vi "ReadSpreadsheetFile.vi"(0 "file (use dialog)":path) -> (1 "Array":dbl[][](array[numeric]), 2 "cancelled":bool, 3 "error out":errorcluster)   [LabVIEW 2012]
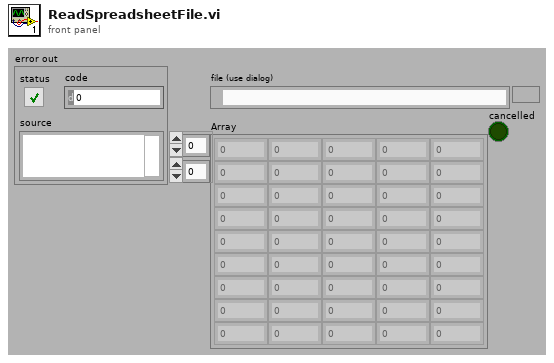
[diagram p1: front panel]
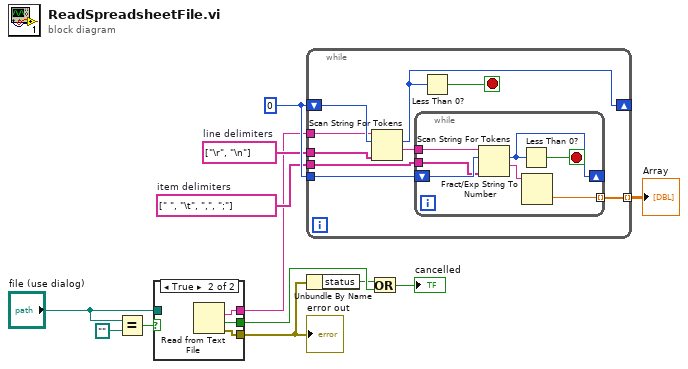
[diagram p0: block diagram]
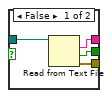
[diagram p2: hidden frame]
diagram:
  w10 = string[] [" ", "\t", ",", ";"]  # item delimiters
  w11 = string[] ["\r", "\n"]  # line delimiters
  w12 = 0 ("offset past token")
  n1 = Equal?(x="file (use dialog)", y=path "") -> (x = y?=w5:bool)
  n2 = case shown="True" w5 {
    tunnel: [w15 w19] -> w8
    tunnel: [w14 w18] -> w2
    tunnel: "file (use dialog)" -> [w16 _]
    tunnel: [w13 w17] -> w4
    frame False {
      n3 = Read from Text File(file (use dialog)=w16) -> (text=w15:string, cancelled=w13:bool, error out=w14:errorcluster)  [unwired: 3 in, 1 out]
    }
    frame True {
      n4 = Read from Text File() -> (text=w19:string, cancelled=w17:bool, error out=w18:errorcluster)  [unwired: 4 in, 1 out]
    }
  }
  "error out" <- w2
  n5 = while {
    shift-right: [w21] -> _
    shift-left: w12 -> [w28]
    tunnel: w11 -> [w27]
    tunnel: w10 -> [w26]
    tunnel: w12 -> [w23]
    tunnel: w8 -> [w22]
    tunnel: [w20] -> w9 mode=indexing
    stop <- w24 stop-if-true
    n6 = Scan String For Tokens(6:w27, 8:w28, 9:w22) -> (1:w25:string, 2:w21:i32)  [unwired: 3 in, 2 out]
    n7 = while {
      shift-right: [w31] -> _
      shift-left: w23 -> [w35]
      tunnel: w26 -> [w34]
      tunnel: w25 -> [w33]
      tunnel: [w30] -> w20 mode=indexing
      stop <- w32 stop-if-true
      n8 = Scan String For Tokens(6:w34, 8:w35, 9:w33) -> (1:w29:string, 2:w31:i32)  [unwired: 3 in, 2 out]
      n9 = Less Than 0?(x=w31) -> (x < 0?=w32:bool)
      n10 = Fract/Exp String To Number(string=w29) -> (number=w30:dbl)  [unwired: 3 in, 1 out]
    }
    n11 = Less Than 0?(x=w21) -> (x < 0?=w24:bool)
  }
  "Array" <- w9
  n12 = Unbundle By Name(w2) -> ("status"=w1:bool)
  n13 = Or(x=w1, y=w4) -> (x .or. y?=→"cancelled":bool)
